vi "Detector Setup.vi"(8 "error in (no error)":errorcluster, 11 "PRIME Detector in":refnum<class "PRIME Detector.lvclass">) -> (0 "error out":errorcluster, 2 "Detector Config.Detector":u16, 3 "PRIME Detector out":refnum<class "PRIME Detector.lvclass">)   [LabVIEW 2024, in "PRIME Detector.lvclass"]
uses:
  PRIME Detector.lvclass
  PRIME Detector cluster Status.ctl
  PRIME Detector.lvclass/PRIME Detector.ctl
  ebdf0ea1-bc8f-4ec3-b978-86607bdb800c.vi
  Detector Class.lvclass
panel:
  out "Status":T1
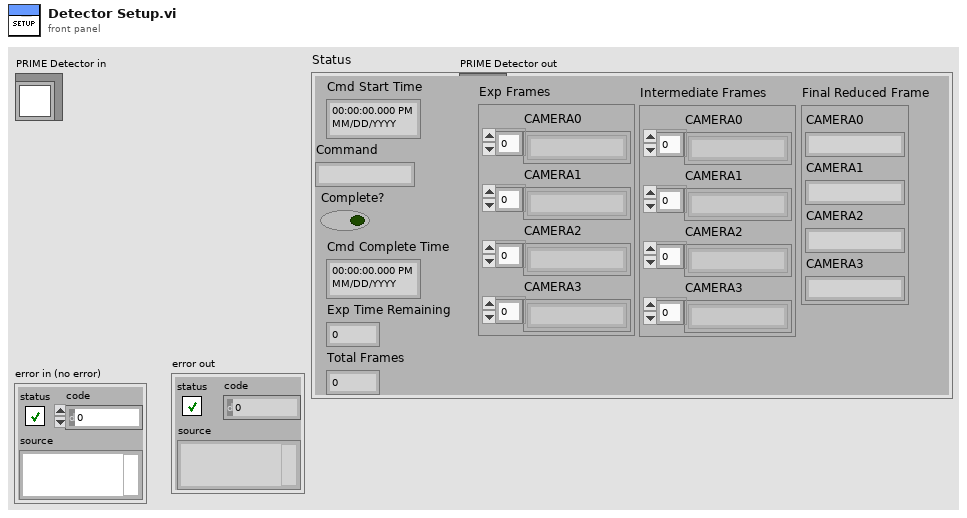
[diagram p1: front panel]
types:
  T1 = typedef "PRIME Detector cluster Status.ctl" = cluster{"Cmd Start Time":timestamp, "Command":string, "Complete?":bool, "Cmd Complete Time":timestamp, "Exp Time Remaining":dbl, "Total Frames":i32, "Exp Frames":cluster{"CAMERA0":string[], "CAMERA1":string[], "CAMERA2":string[], "CAMERA3":string[]}, "Intermediate Frames":cluster{"CAMERA0":string[], "CAMERA1":string[], "CAMERA2":string[], "CAMERA3":string[]}, "Final Reduced Frame":cluster{"CAMERA0":string, "CAMERA1":string, "CAMERA2":string, "CAMERA3":string}}
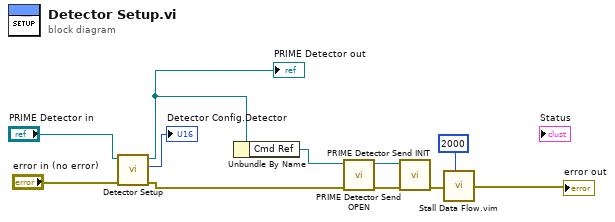
[diagram p0: block diagram]
diagram:
  n1 = call-parent "Detector Setup.vi"("error in (no error)"="error in (no error)", "Detector Class in"="PRIME Detector in") -> ("error out"=w4:errorcluster, "Detector Config.Detector"=→"Detector Config.Detector":u16, "Detector Class out"=w6:refnum<class "PRIME Detector.lvclass">)  [unwired: 7 in]
  "PRIME Detector out" <- w6
  n2 = Unbundle By Name(w6) -> ("Cmd Ref"=w5:refnum<k5>)
  n3 = call "PRIME Detector Send OPEN.vi"("error in (no error)"=w4, "connection ID"=w5) -> ("error out"=w7:errorcluster, "connection ID out"=w8:refnum<k5>)  [unwired: 8 in]
  n4 = call "PRIME Detector Send INIT.vi"("error in (no error)"=w7, "connection ID"=w8) -> ("error out"=w3:errorcluster)  [unwired: 8 in, 1 out]
  n5 = call "Stall Data Flow.vim"("value in"=w3, "milliseconds to wait"=u32 2000) -> ("value out"=→"error out":errorcluster)  [unwired: 1 out]
